vi "Julian Day_with_millisec_BM_subVI.vi"() -> (4 "Julian Day":dbl format="%#_12g", 6 "hour":dbl, 8 "minute":dbl, 10 "second":dbl, 15 "Decimal second":dbl)   [LabVIEW 2021]
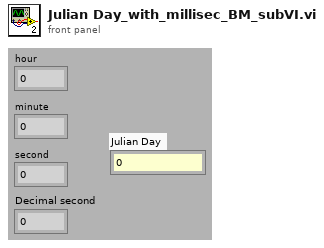
[diagram p1: front panel]
types:
  T1 = cluster{"second":i32, "minute":i32, "hour":i32, "day of month":i32, "month":i32, "year":i32, "day of week":i32, "day of year":i32, "is DST":i32}
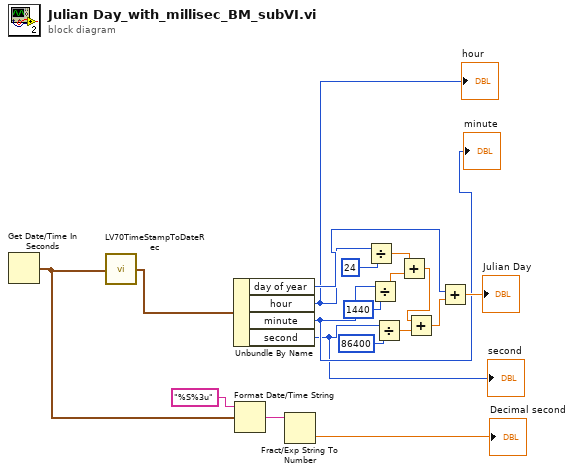
[diagram p0: block diagram]
diagram:
  n1 = Get Date/Time In Seconds() -> (seconds since 1Jan1904=w4:timestamp)
  n2 = call <vilib>:"LV70TimeStampToDateRec.vi"("time stamp"=w4) -> ("date time rec"=w9:T1)
  n3 = Unbundle By Name(w9) -> ("day of year"=w18:i32, "hour"=w7:i32, "minute"=w6:i32, "second"=w5:i32)
  "hour" <- w7
  "minute" <- w6
  "second" <- w5
  n4 = Format Date/Time String(time format string (%c)="%S%3u", seconds (now)=w4) -> (date/time string=w2:string)  [unwired: 1 in]
  n5 = Fract/Exp String To Number(string=w2) -> (number=→"Decimal second":dbl)  [unwired: 3 in, 1 out]
  n6 = Divide(x=w7, y=24) -> (x/y=w15:dbl)
  n7 = Divide(x=w6, y=1440) -> (x/y=w13:dbl)
  n8 = Divide(x=w5, y=86400) -> (x/y=w14:dbl)
  n9 = Add(x=w15, y=w13) -> (x+y=w16:dbl)
  n10 = Add(x=w16, y=w14) -> (x+y=w17:dbl)
  n11 = Add(x=w18, y=w17) -> (x+y=→"Julian Day":dbl)
